vi "Query to KeyValue Pairs.vi"(11 "query":string) -> (3 "Query":cluster{"argument":string, "value":string}[](array[cluster]))   [LabVIEW 2013, in "openURI.lvlib"]
uses:
  openURI.lvlib
  <vilib>/regexp/Match Regular Expression.xnode
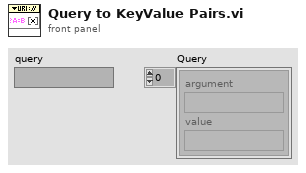
[diagram p1: front panel]
types:
  T1 = cluster{"before match":string, "after match":string}
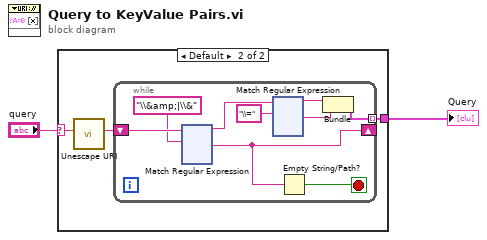
[diagram p0: block diagram]
diagram:
  n1 = case shown="Default" "query" {
    selector: "query" -> [_ w4]
    tunnel: [_ w5] -> w2
    frame "" {
    }
    frame Default {
      n2 = call "Unescape URI.vi"("Escaped URI"=w4) -> ("URI"=w3:string)  [unwired: 10 in]
      n3 = while {
        tunnel: [w9] -> w5 mode=indexing
        shift-right: [w8] -> _
        shift-left: w3 -> [w14]
        stop <- w7 stop-if-true
        n4 = xnode "Match Regular Expression"("input string"=w14, "regular expression"="\\&amp;|\\&") -> ("before match"=w12:string, "after match"=w8:string)  [unwired: 4 in, 3 out]
        n5 = xnode "Match Regular Expression"("input string"=w12, "regular expression"="\\=") -> ("before match"=w11:string, "after match"=w10:string)  [unwired: 4 in, 3 out]
        n6 = Empty String/Path?(string/path=w8) -> (empty?=w7:bool)
        n7 = Bundle("before match"=w11, "after match"=w10) -> (w9:T1)  [unwired: 1 in]
      }
    }
  }
  "Query" <- w2
